vi "unflattenTimeFromXML_Array.vi"(8 "error in (no error)":errorcluster, 9 "timeUnitInXML":T1, 10 "xmlString":string, 11 "timeForType":dbl[unit][](array[numeric])=[15.707963267948964, 31.415926535897928, 47.12388980384689, 62.831853071795855]) -> (0 "error out":errorcluster, 3 "time":dbl[unit][](array[numeric]))   [LabVIEW 2012, in "UnitsAndXML.lvlib"]
uses:
  <userlib>/Common/UnitsAndXML/UnitsAndXML.lvlib
  <userlib>/Common/UnitsAndXML/FlattenItemWithUnitToXML/FlattenTimeToXML/TimeUnit.ctl
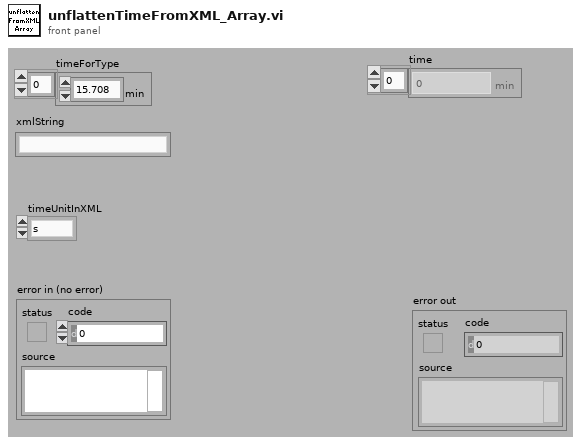
[diagram p1: front panel]
types:
  T1 = typedef "UnitsAndXML.lvlib/TimeUnit.ctl" = enum16{"s", "d", "h", "min", "a"}
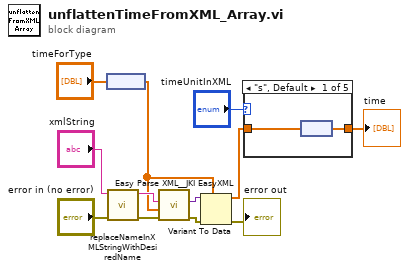
[diagram p0: block diagram]
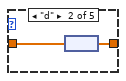
[diagram p2: hidden frame]
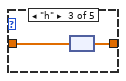
[diagram p3: hidden frame]
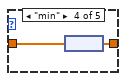
[diagram p4: hidden frame]
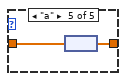
[diagram p5: hidden frame]
diagram:
  n1 = node("timeForType") -> (w9:dbl[])
  n2 = call <userlib>:"replaceNameInXMLStringWithDesiredName.vi"("error in"="error in (no error)", "xmlString"="xmlString") -> ("error out"=w4:errorcluster, "revisedXMLString"=w10:string)  [unwired: 8 in]
  n3 = call <vilib>:"Easy Parse XML__JKI EasyXML.vi"("error in (no error)"=w4, "LabVIEW Data (Type)"=w9, "XML String"=w10) -> ("error out"=w7:errorcluster, "LabVIEW Data"=w12:variant)  [unwired: 7 in]
  n4 = Variant To Data(error in=w7, type=w9, Variant=w12) -> (data=w2:dbl[], error out=→"error out":errorcluster)
  n5 = case shown="\"s\", Default" "timeUnitInXML" {
    tunnel: w2 -> [w14 w16 w18 w20 w22]
    tunnel: [w13 w15 w17 w19 w21] -> w1
    frame "s", Default {
      n6 = node(w14) -> (w13:dbl[unit][])
    }
    frame "d" {
      n7 = node(w16) -> (w15:dbl[unit][])
    }
    frame "h" {
      n8 = node(w18) -> (w17:dbl[unit][])
    }
    frame "min" {
      n9 = node(w20) -> (w19:dbl[unit][])
    }
    frame "a" {
      n10 = node(w22) -> (w21:dbl[unit][])
    }
  }
  "time" <- w1
